vi "HTTPPost.vi"(4 "Front Panel References":refnum<vi>[](array[refnum]), 5 "Season Log":string, 6 "Clock Type":T1, 7 "Budget Year RID":string="5", 8 "error in (no error)":errorcluster, 9 "Student RID":string, 10 "usertoken":string="b287yg_uyp_dsagzw8b755gx7bvr8hfmdp3fu53", 11 "tableID":string="bmu8iv63w") -> (0 "error out":errorcluster, 2 "body":string, 3 "headers":string)   [LabVIEW 2017]
uses:
  Controls/ClockType.ctl
  <vilib>/httpClient/POSTBuffer.vi
  <vilib>/httpClient/LabVIEWHTTPClient.lvlib
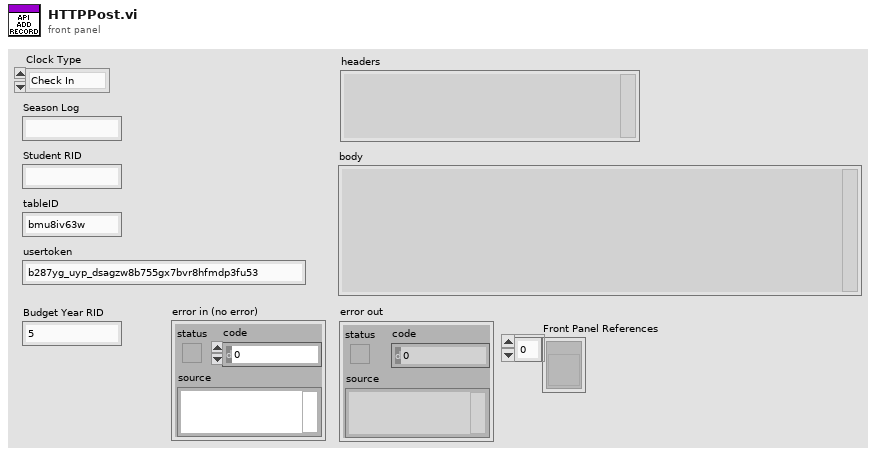
[diagram p1: front panel]
types:
  T1 = typedef "ClockType.ctl" = enum16{"Check In", "Check Out"}
  T2 = enum8{"Enabled", "Disabled", "Disabled and Grayed Out"}
  T3 = typedef "LabVIEWHTTPClient.lvlib/ClientHandle.ctl" = refnum<k1>
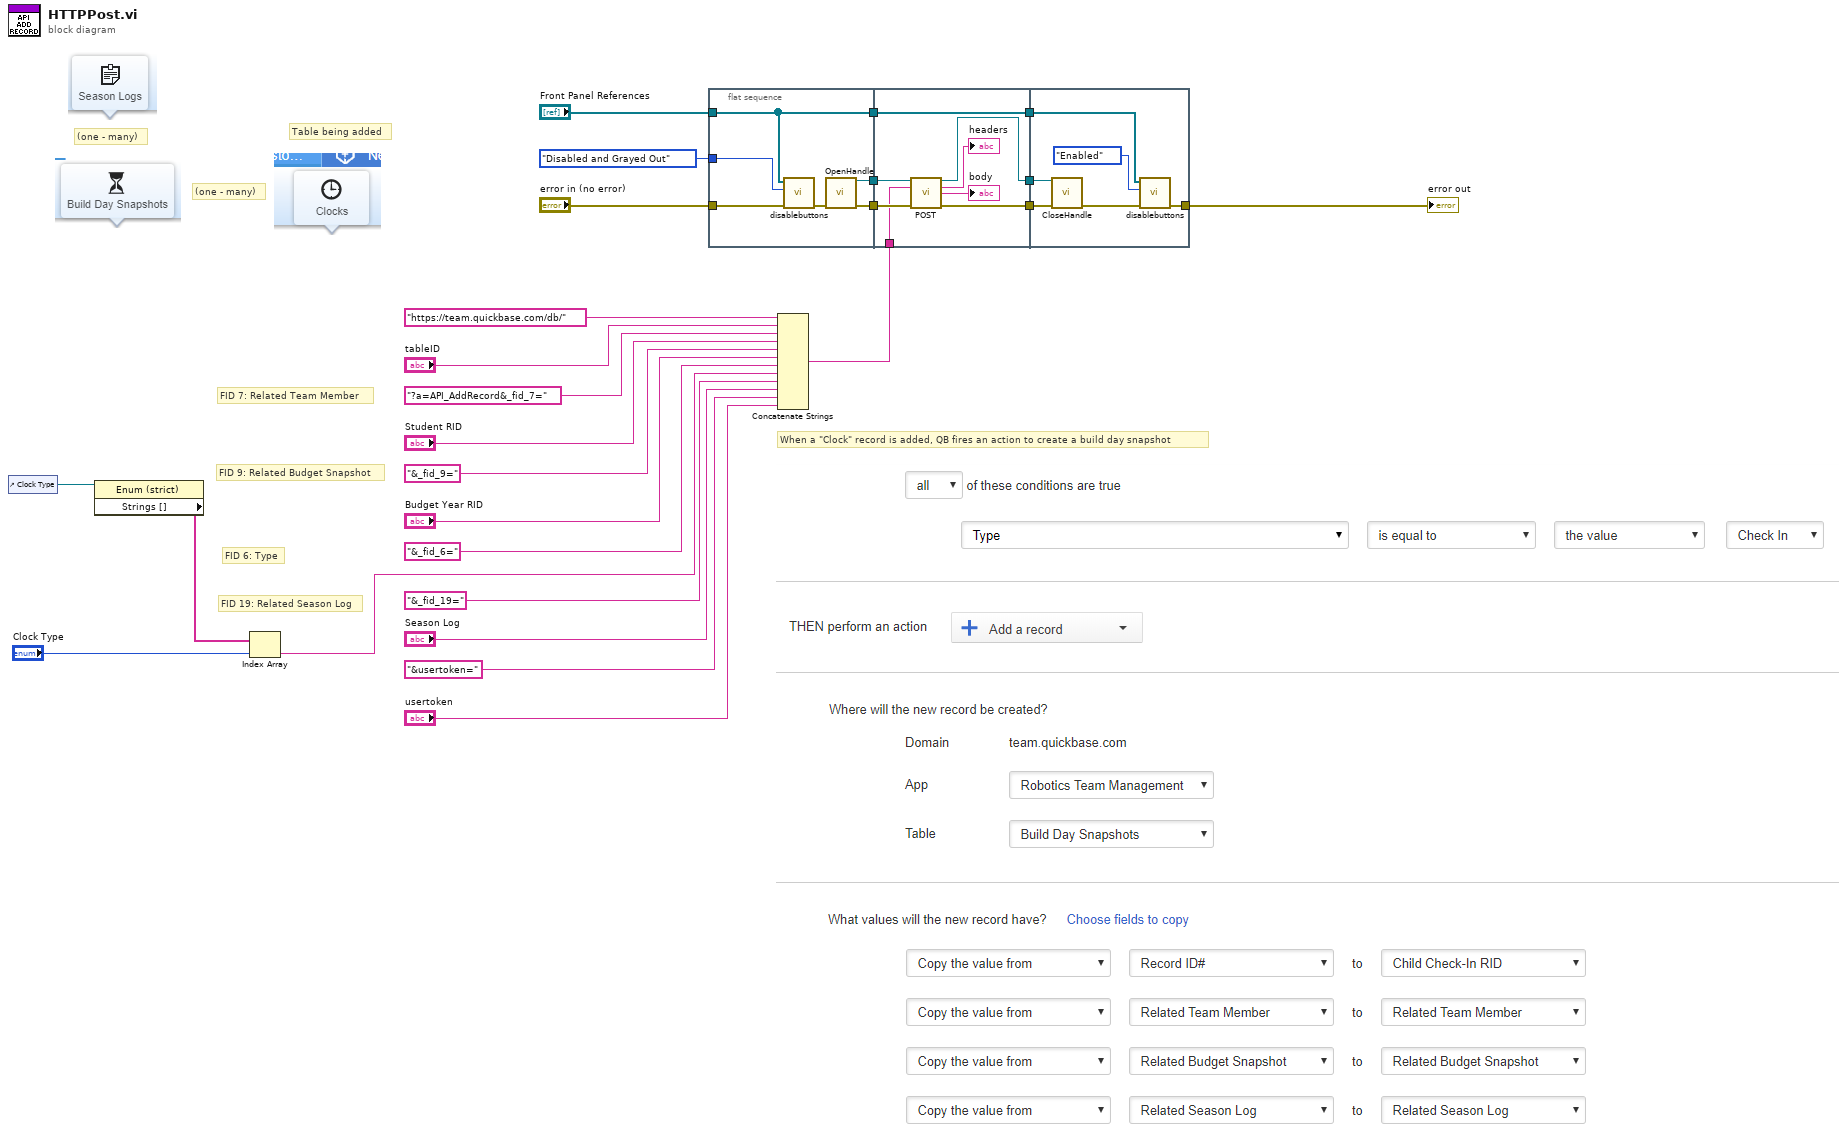
[diagram p0: block diagram]
diagram:
  # "When a \"Clock\" record is added, QB fires an action to create a build day snapshot"
  # "FID 19: Related Season Log"
  # "FID 6: Type"
  # "FID 7: Related Team Member"
  # "FID 9: Related Budget Snapshot"
  # "(one - many)"
  # "(one - many)"
  # "Table being added"
  n1 = control-ref of="Clock Type"() -> (w18:refnum<vi>)
  n2 = property class="Enum (strict)"(reference=w18) -> ("Strings []"=w17:string[])  [unwired: 1 in, 2 out]
  n3 = Index Array(array=w17, index="Clock Type") -> (element=w16:string)
  n4 = flat-sequence {
    tunnel: "error in (no error)" -> [w30]
    tunnel: [w32] -> w11
    tunnel: [w31] -> w10
    tunnel: T2."Disabled and Grayed Out" ("Disabled") -> [w28]
    tunnel: "Front Panel References" -> [w27]
    tunnel: [w27] -> w6
    tunnel: w22 -> [w33]
    tunnel: [w40] -> w14
    tunnel: [w39] -> w13
    tunnel: w11 -> [w36]
    tunnel: w10 -> [w35]
    tunnel: [w34] -> w7
    tunnel: w6 -> [w34]
    tunnel: w14 -> [w46]
    tunnel: w13 -> [w45]
    tunnel: [w41] -> w5
    tunnel: w7 -> [w44]
    frame #0 {
      n5 = call "disablebuttons.vi"("error in (no error)"=w30, "Disabled"=w28, "Front Panel References"=w27) -> ("error out"=w29:errorcluster)  [unwired: 8 in]
      n6 = call <vilib>:"OpenHandle.vi"("error in (no error)"=w29) -> ("client handle out"=w31:T3, "error out"=w32:errorcluster)  [unwired: 13 in]
    }
    frame #1 {
      n7 = call-poly <vilib>:"POST.vi"("client handle"=w35, "url"=w33, "error in (no error)"=w36) -> ("client handle out"=w40:T3, "headers"=→"headers":string, "body"=→"body":string, "error out"=w39:errorcluster)  [unwired: 9 in]
    }
    frame #2 {
      n8 = call <vilib>:"CloseHandle.vi"("client handle"=w46, "error in (no error)"=w45) -> ("error out"=w42:errorcluster)  [unwired: 13 in]
      n9 = call "disablebuttons.vi"("error in (no error)"=w42, "Disabled"=T2."Enabled", "Front Panel References"=w44) -> ("error out"=w41:errorcluster)  [unwired: 8 in]
    }
  }
  n10 = Concatenate Strings("https://team.quickbase.com/db/" ("string"), "tableID", "?a=API_AddRecord&_fid_7=" ("string"), "Student RID", "&_fid_9=" ("string"), "Budget Year RID", "&_fid_6=" ("string"), w16, "&_fid_19=" ("string"), "Season Log", "&usertoken=" ("string"), "usertoken") -> (w22:string)
  "error out" <- w5
